vi "Write Multi Data.vi"(7 "Alias":string, 8 "error in (no error)":errorcluster, 9 "Data Alias Array":string[](array[string]), 10 "Data Array":refnum<class "Data.lvclass">[](array[class]), 11 "Multi Data in":refnum<class "Multi Data.lvclass">) -> (0 "error out":errorcluster, 3 "Multi Data out":refnum<class "Multi Data.lvclass">)   [LabVIEW 2020, in "Publisher.lvlib" / "Multi Data.lvclass"]
doc: "Populate the class."
uses:
  Multi Data.lvclass
  PPL/HDH.Data.Generic.lvlibp/Data.lvclass
  Multi Data.lvclass/Multi Data.ctl
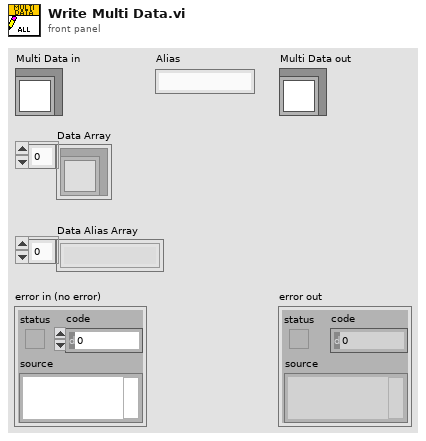
[diagram p1: front panel]
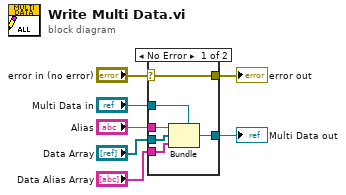
[diagram p0: block diagram]
diagram:
  n1 = case shown="No Error" "error in (no error)" {
    selector: "error in (no error)" -> [w13 w14]
    tunnel: [w13 w14] -> w6
    tunnel: [w11 w15] -> w4
    tunnel: "Multi Data in" -> [w12 w15]
    tunnel: "Alias" -> [w10 _]
    tunnel: "Data Array" -> [w9 _]
    tunnel: "Data Alias Array" -> [w8 _]
    frame No Error {
      n2 = Bundle(cluster=w12, w10, w9, w8) -> (w11:refnum<class "Multi Data.lvclass">)
    }
    frame Error {
    }
  }
  "error out" <- w6
  "Multi Data out" <- w4
